vi "GageAcquLoop_Double.vi"(5 "GageParams.":T1={"Mode"=0, "Depth"=1024.0, "Segments"=1024, "Channel"=0} {"Mode" items=["Normal (0)"=0, "HWAverage (2)"=2, "MultiRecord (16)"=16]}, 7 "Refs.":T2, 8 "error in":errorcluster, 9 "SignalOut":refnum<queue>, 11 "GageCtrl":refnum<queue>) -> (0 "error out":errorcluster)   [LabVIEW 2013]
uses:
  Gage_States.ctl
  ControlDef/Signal.ctl
  ControlDef/QuitProg.vi
  InstruGloble.vi
  ProcessMethods/SignalAverager/ProcessStates.ctl
  ProcessMethods/SignalAverager/DAQParams.ctl
  <instrlib>/ESP300/Public/Position_ESP300.vi
  <instrlib>/ESP300/ESP300.lvlib
  <instrlib>/Micos_uic/Public/Position_Micos.vi
  <instrlib>/Micos_uic/Micos_uic.lvlib
  GageAcqu.Refs.ctl
  GageParams.ctl
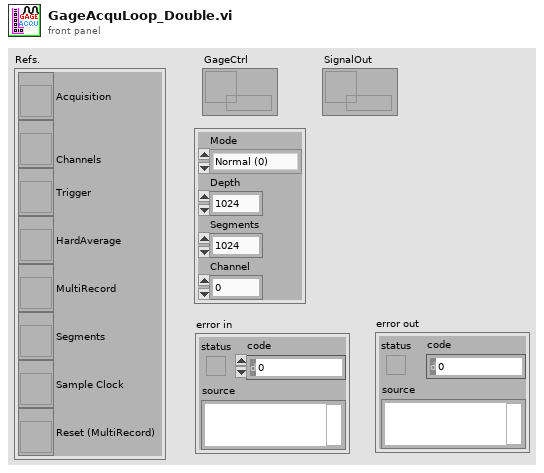
[diagram p1: front panel]
types:
  T1 = typedef "GageParams.ctl" = cluster{"Mode":u16, "Depth":dbl, "Segments":u32, "Channel":u16}
  T2 = typedef "GageAcqu.Refs.ctl" = cluster{"Acquisition":refnum<vi>, "Channels":refnum<vi>, "Trigger":refnum<vi>, "HardAverage":refnum<vi>, "MultiRecord":refnum<vi>, "Segments":refnum<vi>, "Sample Clock":refnum<vi>, "Reset (MultiRecord)":refnum<vi>}
  T3 = typedef "Gage_States.ctl" = enum16{"Initialize", "Config, Commit, Start", "Wait Idle", "Transfer", "CloseSystem"}
  T4 = cluster{"Handle":u32, "Sample size":u32, "Resolution":i32, "Offset":i32, "Channels":u32, "Boards":u32}
  T5 = typedef "Signal.ctl" = cluster{"Command":T6, "Params":variant}
  T6 = typedef "ProcessStates.ctl" = enum16{"Initialize", "Normal", "Display", "Write2Buffer", "CalcMzArray", "StartSave", "StopSave", "ConfigChanged", "EndOfLine", "SetFilterParams", "SetGraphsEnable", "SetAcquisitionParams", "ChangeDisplayIncrement", "ChangeRepRate", "SetWriterRef", "Quit", "StartOfLine"}
  T7 = typedef "DAQParams.ctl" = cluster{"TrigDelay":dbl, "Offset":i32, "Resolution":i32, "Range (mV)":u32, "Sample Rate":dbl, "Depth":dbl, "Segments":u32}
  T8 = cluster{"Handle":u32, "Sample Size":u32, "Resolution":i32, "Offset":i32, "Channels":u32, "Boards":u32}
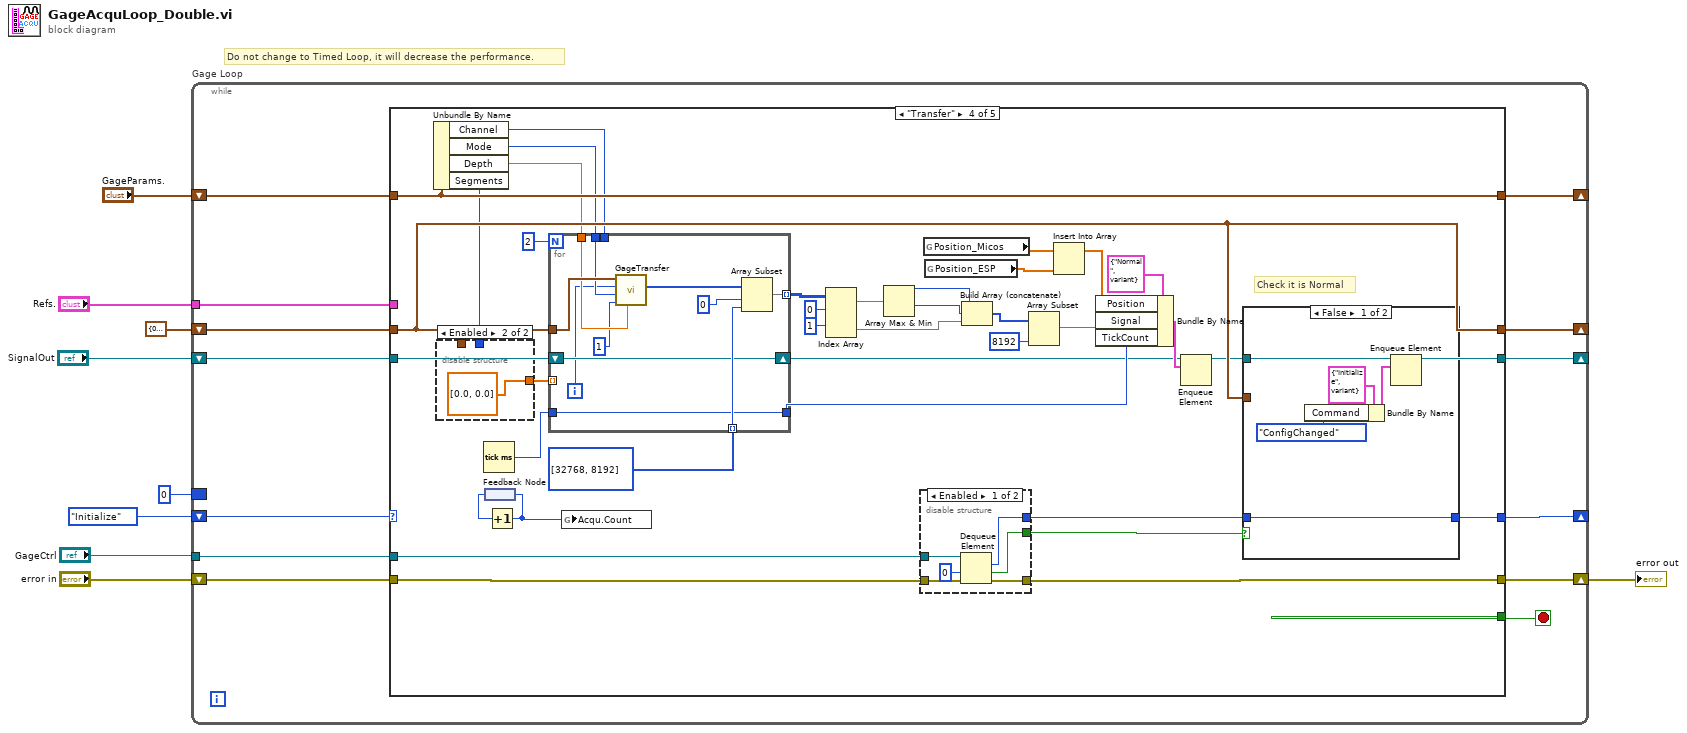
[diagram p0: block diagram]
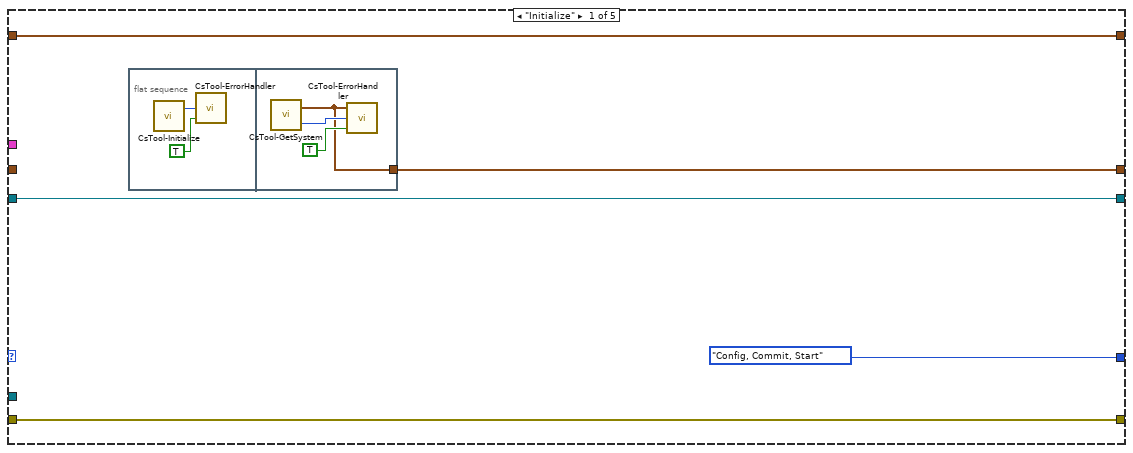
[diagram p2: hidden frame]
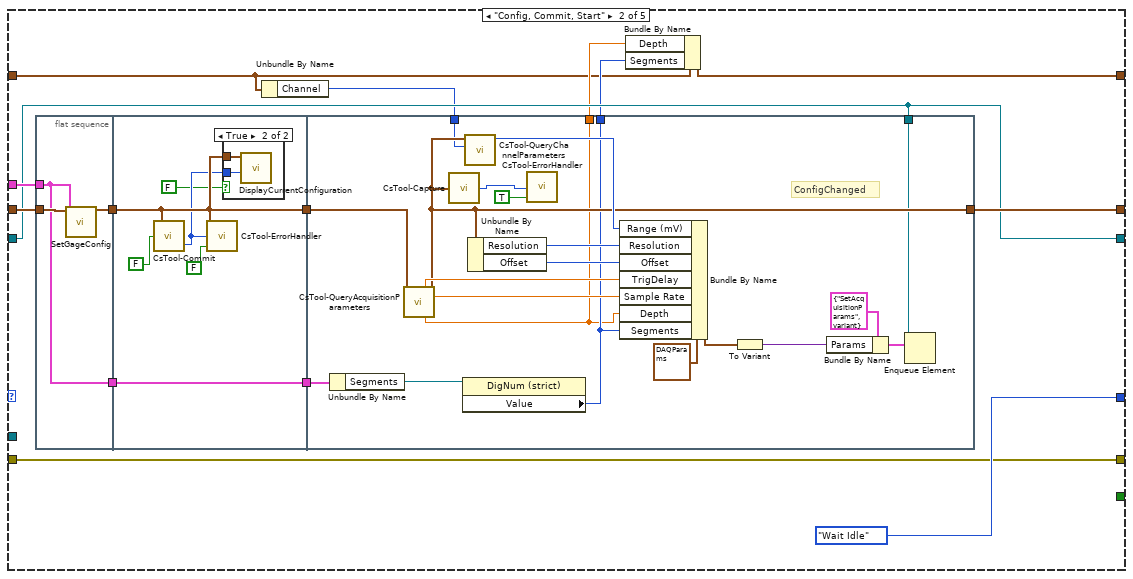
[diagram p3: hidden frame]
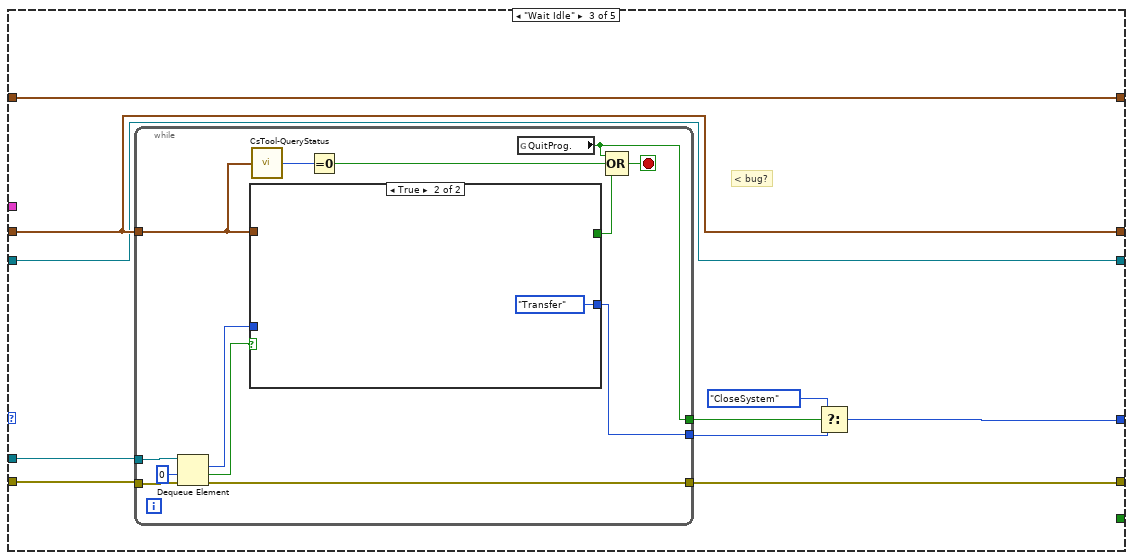
[diagram p5: hidden frame]
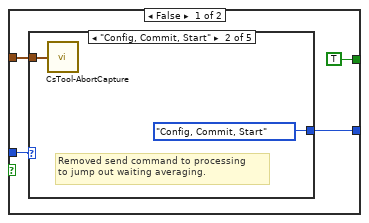
[diagram p6: hidden frame]
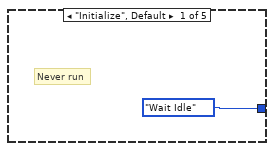
[diagram p7: hidden frame]
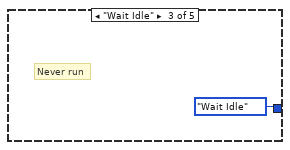
[diagram p8: hidden frame]
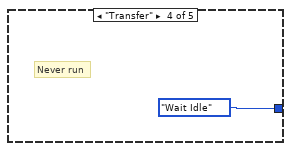
[diagram p9: hidden frame]
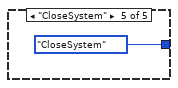
[diagram p10: hidden frame]
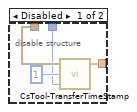
[diagram p11: hidden frame]
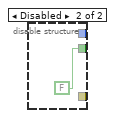
[diagram p12: hidden frame]
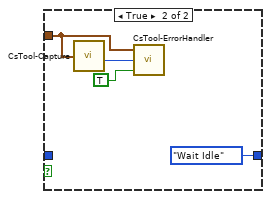
[diagram p13: hidden frame]
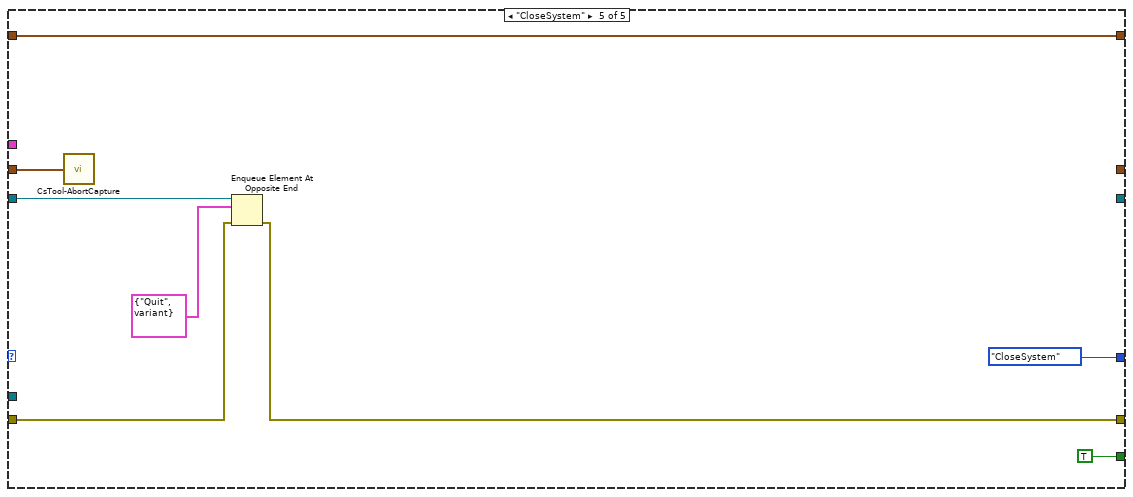
[diagram p14: hidden frame]
diagram:
  # "Do not change to Timed Loop, it will decrease the performance."
  n1 = while "Gage Loop" {
    shift-right: [w21] -> _
    shift-left: Gage_States."Initialize" ("Gage States") -> [w10]
    shift-right: [w20] -> _
    shift-left: "SignalOut" -> [w22]
    shift-right: [w18] -> _
    shift-left: T4 {"Handle"=0, "Sample size"=0, "Resolution"=0, "Offset"=0, "Channels"=0, "Boards"=0} ("Handle Cluster") -> [w19]
    border: u32 0 ("Numeric") -> [_]
    tunnel: "GageCtrl" -> [w16]
    shift-right: [w14] -> w3
    shift-left: "error in" -> [w15]
    tunnel: "Refs." -> [w13]
    shift-right: [w12] -> _
    shift-left: "GageParams." -> [w11]
    stop <- w17 stop-if-true
    n2 = case shown="\"Transfer\"" w10 {
      tunnel: w22 -> [w26 w40 w83 w148 w185]
      tunnel: [Gage_States."Config, Commit, Start" ("DAQ Status") Gage_States."Wait Idle" ("DAQ Status") w82 w143 Gage_States."CloseSystem" ("DAQ Status")] -> w21
      tunnel: [w26 w40 w83 w124 _] -> w20
      tunnel: w19 -> [_ w45 w87 w147 w187]
      tunnel: [w25 w44 w87 w147 _] -> w18
      tunnel: [_ _ _ _ TRUE] -> w17
      tunnel: w16 -> [_ _ w86 w146 _]
      tunnel: w15 -> [w24 w46 w85 w145 w183]
      tunnel: [w24 w46 w84 w144 w182] -> w14
      tunnel: w13 -> [_ w41 _ _ _]
      tunnel: [w23 w37 w79 w142 w184] -> w12
      tunnel: w11 -> [w23 w34 w79 w142 w184]
      frame "Initialize" {
        n3 = flat-sequence {
          tunnel: [w30] -> w25
          frame #0 {
            n4 = call <instrlib>:"CsTool-Initialize.vi"() -> ("Number Of Systems"=w29:i32)  [unwired: 1 out]
            n5 = call <instrlib>:"CsTool-ErrorHandler.vi"("StopOnError (true)"=TRUE, "Error Code"=w29) -> ()  [unwired: 1 in, 1 out]
          }
          frame #1 {
            n6 = call <instrlib>:"CsTool-GetSystem.vi"() -> ("Error Code"=w32:i32, "Handle Cluster"=w30:T4)  [unwired: 4 in]
            n7 = call <instrlib>:"CsTool-ErrorHandler.vi"("StopOnError (true)"=TRUE, "Error Code"=w32, "Handle Cluster"=w30) -> ()  [unwired: 1 out]
          }
        }
      }
      frame "Config, Commit, Start" {
        n8 = flat-sequence {
          tunnel: w45 -> [w49]
          tunnel: [w49] -> w43
          tunnel: w41 -> [w48]
          tunnel: [w48] -> w39
          tunnel: w43 -> [w53]
          tunnel: [w53] -> w42
          tunnel: w39 -> [w50]
          tunnel: [w50] -> w38
          tunnel: w42 -> [w75]
          tunnel: [w71] -> w44
          tunnel: w40 -> [w66]
          tunnel: w38 -> [w62]
          tunnel: [w60] -> w36
          tunnel: [w59] -> w35
          tunnel: w33 -> [w58]
          frame #0 {
            n9 = call "SetGageConfig.vi"("Gage Acqu."=w48, "Handle Cluster"=w49) -> ()  [unwired: 10 in]
          }
          frame #1 {
            n10 = call <instrlib>:"CsTool-Commit.vi"("Coerce Flag (f)"=FALSE, "Handle Cluster"=w53) -> ("Error Code"=w52:i32)  [unwired: 1 in, 1 out]
            n11 = call <instrlib>:"CsTool-ErrorHandler.vi"("StopOnError (true)"=FALSE, "Error Code"=w52, "Handle Cluster"=w53) -> ()  [unwired: 1 out]
            n12 = case shown="True" FALSE {
              tunnel: w53 -> [_ w57]
              tunnel: w52 -> [_ w56]
              frame False {
              }
              frame True {
                n13 = call <instrlib>:"DisplayCurrentConfiguration.vi"("error code  in"=w56, "Handle Cluster"=w57) -> ()  [unwired: 10 in]
              }
            }
          }
          frame #2 {
            # "ConfigChanged"
            n14 = Unbundle By Name(w62) -> ("Segments"=w61:refnum<vi>)
            n15 = call <instrlib>:"CsTool-QueryAcquisitionParameters.vi"("Handle Cluster"=w75) -> ("Trigger Delay"=w73:dbl, "Output Handle Cluster"=w71:T8, "Sample Rate"=w72:dbl, "Depth"=w59:dbl)  [unwired: 4 in, 7 out]
            n16 = call <instrlib>:"CsTool-Capture.vi"("Handle Cluster"=w71) -> ("Error Code"=w77:i32)
            n17 = property class="DigNum (strict)"(reference=w61) -> ("Value"=w60:u32)  [unwired: 1 in, 2 out]
            n18 = call <instrlib>:"CsTool-QueryChannelParameters.vi"("Handle Cluster"=w71, "Channel"=w58) -> ("Range (mV)"=w74:u32)  [unwired: 7 out]
            n19 = Unbundle By Name(w71) -> ("Resolution"=w70:i32, "Offset"=w69:i32)
            n20 = call <instrlib>:"CsTool-ErrorHandler.vi"("StopOnError (true)"=TRUE, "Error Code"=w77) -> ()  [unwired: 1 in, 1 out]
            n21 = Bundle By Name(cluster=T7 {"TrigDelay"=0.0, "Offset"=0, "Resolution"=-32768, "Range (mV)"=0, "Sample Rate"=100000000.0, "Depth"=16384.0, "Segments"=1} ("Value"), "Range (mV)"=w74, "Resolution"=w70, "Offset"=w69, "TrigDelay"=w73, "Sample Rate"=w72, "Depth"=w59, "Segments"=w60) -> (w64:T7)
            n22 = To Variant(anything=w64) -> (Variant=w63:variant)
            n23 = Bundle By Name(cluster=T5 {"Command"=enum."SetAcquisitionParams", "Params"=variant} ("element"), "Params"=w63) -> (w65:T5)
            n24 = Enqueue Element(queue=w66, element=w65) -> ()  [unwired: 2 in, 3 out]
          }
        }
        n25 = Unbundle By Name(w34) -> ("Channel"=w33:u16)
        n26 = Bundle By Name(cluster=w34, "Depth"=w35, "Segments"=w36) -> (w37:T1)
      }
      frame "Wait Idle" {
        # "< bug?"
        n27 = while "To get highest repetive rate,change waiting time to 0." {
          tunnel: w87 -> [w90]
          tunnel: w86 -> [w96]
          tunnel: w85 -> [w95]
          tunnel: [w92] -> w84
          tunnel: [w91] -> w81
          tunnel: [w88] -> w78
          stop <- w98 stop-if-true
          n28 = Dequeue Element(queue=w96, timeout in ms (-1)=0, error in (no error)=w95) -> (element=w94:T3, timed out?=w93:bool, error out=w92:errorcluster)  [unwired: 1 out]
          n29 = case shown="True" w93 {
            tunnel: [TRUE _] -> w97
            tunnel: w94 -> [w104 _]
            tunnel: [w103 Gage_States."Transfer" ("DAQ Status 2")] -> w91
            tunnel: w90 -> [w101 _]
            frame False {
              n30 = case shown="\"Config, Commit, Start\"" w104 {
                tunnel: [Gage_States."Wait Idle" ("t") Gage_States."Config, Commit, Start" ("t") Gage_States."Wait Idle" ("t") Gage_States."Wait Idle" ("t") Gage_States."CloseSystem" ("t")] -> w103
                tunnel: w101 -> [_ w106 _ _ _]
                frame "Initialize", Default {
                  # "Never run"
                }
                frame "Config, Commit, Start" {
                  # "Removed send command to processing\nto jump out waiting averaging."
                  n31 = call <instrlib>:"CsTool-AbortCapture.vi"("Handle Cluster"=w106) -> ()  [unwired: 1 out]
                }
                frame "Wait Idle" {
                  # "Never run"
                }
                frame "Transfer" {
                  # "Never run"
                }
                frame "CloseSystem" {
                }
              }
            }
            frame True {
            }
          }
          n32 = call <instrlib>:"CsTool-QueryStatus.vi"("Handle Cluster"=w90) -> ("Status"=w100:i32)
          n33 = Equal To 0?(x=w100) -> (x = 0?=w99:bool)
          n34 = global read "QuitProg.vi" "QuitProg."() -> (w88:bool)
          n35 = Compound Arithmetic op=OR(w88, w99, w97) -> (w98:bool)
        }
        n36 = Select(t=Gage_States."CloseSystem", s=w78, f=w81) -> (s? t:f=w82:T3)
      }
      frame "Transfer" {
        # "Check it is Normal"
        n37 = Unbundle By Name(w142) -> ("Channel"=w134:u16, "Mode"=w133:u16, "Depth"=w141:dbl, "Segments"=w135:u32)
        n38 = disable-structure shown="Enabled" {
          disable-tunnel: w147 -> [w152 _]
          disable-tunnel: [w150 dbl[] [0.0, 0.0]] -> w136
          disable-tunnel: w135 -> [w149 _]
          frame Disabled {
            n39 = call <instrlib>:"CsTool-TransferTimeStamp.vi"("Length (1)"=w149, "Segment (1)"=u32 1, "Handle Cluster"=w152) -> ("TS Time"=w150:dbl[])  [unwired: 2 out]
          }
          frame Enabled {
          }
        }
        n40 = Tick Count (ms)() -> (millisecond timer value=w132:u32)
        n41 = feedback #1() -> (w140:u32)
        n42 = Increment(x=w140) -> (x+1=w139:u32)
        n43 = feedback-in #1(w139) -> ()
        n44 = for {
          N: 2 -> [_]
          tunnel: w147 -> [w164]
          tunnel: w141 -> [w162]
          shift-right: [w158] -> w122
          shift-left: w148 -> [w158]
          tunnel: w136 -> [_] mode=indexing
          tunnel: w134 -> [_]
          tunnel: w133 -> [w161]
          tunnel: w132 -> [w157]
          tunnel: i32[] [32768, 8192] -> [w159] mode=indexing
          tunnel: [w157] -> w123
          tunnel: [w156] -> w121 mode=indexing
          i -> [w155]
          n45 = call "GageTransfer.vi"("Length (4096)"=w162, "Segment (1)"=u32 1, "Mode (0)"=w161, "Channel (0)"=w155, "Handle Cluster"=w164) -> ("Data_Raw"=w163:i32[])  [unwired: 3 in, 3 out]
          n46 = Array Subset(array=w163, index=0, length=w159) -> (w156:i32[])
        }
        n47 = global write "InstruGloble.vi" "Acqu.Count"(w139) -> ()
        n48 = Index Array(array=w121, index (row) #1=0 ("index (row)"), index (row) #2=1 ("index (row)")) -> (element #1=w116:i32[], element #2=w118:i32[])  [unwired: 2 in]
        n49 = Array Max & Min(array=w116) -> (max value=w114:i32, min value=w115:i32)  [unwired: 2 out]
        n50 = disable-structure shown="Enabled" {
          disable-tunnel: w146 -> [w170 _]
          disable-tunnel: w145 -> [w169 _]
          disable-tunnel: [w168 _] -> w144
          disable-tunnel: [w167 FALSE ("timed out?")] -> w138
          disable-tunnel: [w166 _] -> w137
          frame Enabled {
            n51 = Dequeue Element(queue=w170, timeout in ms (-1)=0, error in (no error)=w169) -> (element=w166:T3, timed out?=w167:bool, error out=w168:errorcluster)  [unwired: 1 out]
          }
          frame Disabled {
          }
        }
        n52 = global read "Position_Micos.vi" "Position_Micos"() -> (w125:dbl[])
        n53 = global read "Position_ESP300.vi" "Position_ESP"() -> (w127:dbl[])
        n54 = Build Array (concatenate)(w114, w115, w118) -> (w117:i32[])
        n55 = Array Subset(array=w117, length=8192) -> (w113:i32[])  [unwired: 1 in]
        n56 = Insert Into Array(array=w125, new element=w127) -> (w126:dbl[])  [unwired: 1 in]
        n57 = Bundle By Name(cluster=T5 {"Command"=enum."Normal", "Params"=variant} ("blank signal"), "Position"=w126, "Signal"=w113, "TickCount"=w123) -> (w128:T5)
        n58 = Enqueue Element(queue=w122, element=w128) -> (queue out=w124:refnum<queue>)  [unwired: 2 in, 2 out]
        n59 = case shown="False" w138 {
          tunnel: w147 -> [_ w178]
          tunnel: w137 -> [w176 _]
          tunnel: [w176 Gage_States."Wait Idle" ("Gage States")] -> w143
          tunnel: w124 -> [w174 _]
          frame False {
            n60 = Bundle By Name(cluster=T5 {"Command"=enum."Initialize", "Params"=variant} ("element"), "Command"=ProcessStates."ConfigChanged") -> (w173:T5)
            n61 = Enqueue Element(queue=w174, element=w173) -> ()  [unwired: 2 in, 3 out]
          }
          frame True {
            n62 = call <instrlib>:"CsTool-Capture.vi"("Handle Cluster"=w178) -> ("Error Code"=w180:i32)
            n63 = call <instrlib>:"CsTool-ErrorHandler.vi"("StopOnError (true)"=TRUE, "Error Code"=w180, "Handle Cluster"=w178) -> ()  [unwired: 1 out]
          }
        }
      }
      frame "CloseSystem" {
        n64 = call <instrlib>:"CsTool-AbortCapture.vi"("Handle Cluster"=w187) -> ()  [unwired: 1 out]
        n65 = Enqueue Element At Opposite End(queue=w185, element=T5 {"Command"=enum."Quit", "Params"=variant}, error in (no error)=w183) -> (error out=w182:errorcluster)  [unwired: 1 in, 2 out]
      }
    }
  }
  "error out" <- w3
